vi "Generate Trace for Dropped Message.vi"(9 "Message Name":string) -> ()   [LabVIEW 2020, in "Actor Framework.lvlib"]
doc: "Generates a DETT User Generated Trace for a message object that was sent to an actor but never received because the actor stopped while the message was still in its queue."
uses:
  ActorFramework/Actor Framework.lvlib
  Registration Mode.ctl
  Localized Strings.vi
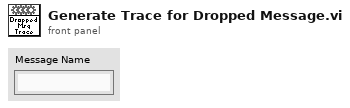
[diagram p1: front panel]
types:
  T1 = typedef "Actor Framework.lvlib/Registration Mode.ctl" = enum16{"Register Actor", "Get ID", "Get Enqueuer", "Deregister Actor", "Get Update Event", "Get All Actors"}
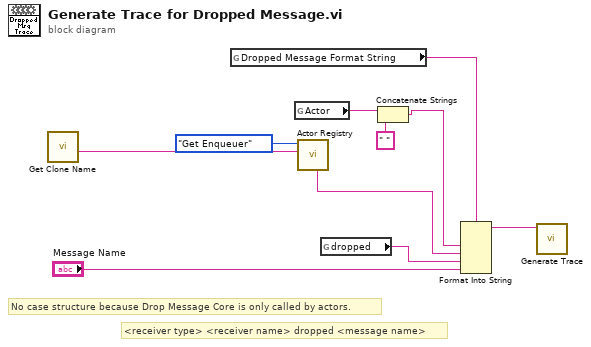
[diagram p0: block diagram]
diagram:
  # "No case structure because Drop Message Core is only called by actors."
  # "<receiver type> <receiver name> dropped <message name>"
  n1 = call "Get Clone Name.vi"() -> ("Clone ID"=w2:string)  [unwired: 10 in, 1 out]
  n2 = global read "Localized Strings.vi" "Dropped Message Format String"() -> (w7:string)
  n3 = global read "Localized Strings.vi" "Actor"() -> (w4:string)
  n4 = call "Actor Registry.vi"("Actor ID"=w2, "Action"=Registration_Mode."Get Enqueuer") -> ("Actor Alias out"=w8:string)  [unwired: 5 in, 4 out]
  n5 = global read "Localized Strings.vi" "dropped"() -> (w6:string)
  n6 = Concatenate Strings(w4, " " ("string")) -> (w9:string)
  n7 = Format Into String(format string=w7, w9, w8, w6, "Message Name") -> (resulting string=w1:string)  [unwired: 2 in, 1 out]
  n8 = call "Generate Trace.vi"("String"=w1) -> ()  [unwired: 11 in]
